vi "TCP_Client.vi"() -> ()   [LabVIEW 2024]
panel:
  in  "Stop Button":bool
  in  "Request":bool
  out "Waveform Graph":dbl[](graph)
  in  "Address":string
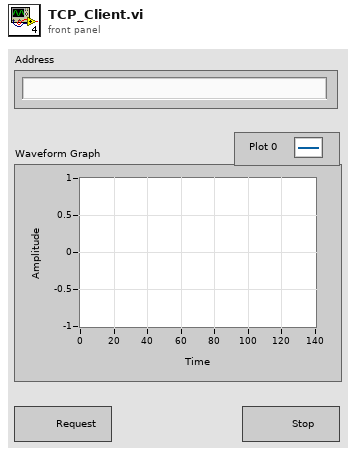
[diagram p1: front panel]
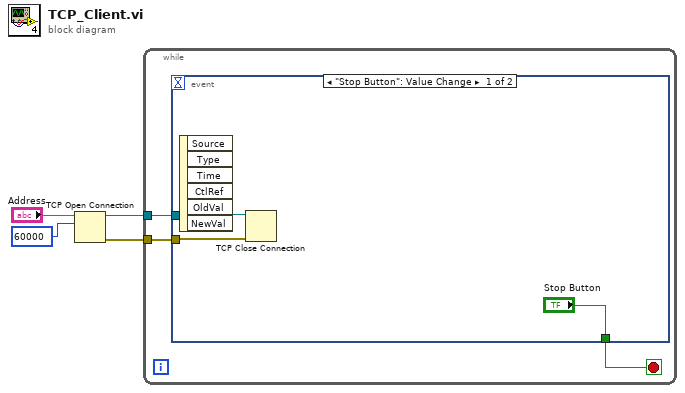
[diagram p0: block diagram]
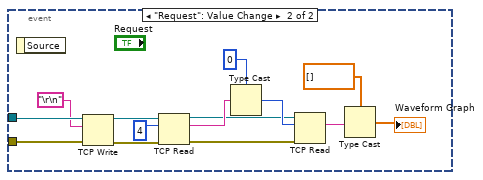
[diagram p2: hidden frame]
diagram:
  n1 = TCP Open Connection(address="Address", remote port or service name=u16 60000) -> (connection ID=w2:refnum<k5>, error out=w1:errorcluster)  [unwired: 3 in]
  n2 = while {
    tunnel: w2 -> [w7]
    tunnel: w1 -> [w6]
    stop <- w5 stop-if-true
    n3 = event shown="[0] \"Stop Button\": Value Change" {
      selector: _ -> [_ _]
      dyn-events: _ -> [_ _]
      timeout: _ -> [_ _]
      tunnel: w7 -> [w9 w24]
      tunnel: w6 -> [w8 w23]
      tunnel: ["Stop Button" _] -> w5
      event "Stop Button": Value Change {
        n4 = event-data() -> ()  [unwired: 1 in, 6 out]
        n5 = TCP Close Connection(connection ID=w9, error in (no error)=w8) -> ()  [unwired: 1 in, 2 out]
      }
      event "Request": Value Change {
        n6 = event-data() -> ()  [unwired: 1 in, 1 out]
        n7 = TCP Write(connection ID=w24, data in="\r\n", error in (no error)=w23) -> (connection ID out=w22:refnum<k5>, error out=w21:errorcluster)  [unwired: 1 in, 1 out]
        n8 = TCP Read(connection ID=w22, bytes to read=4, error in (no error)=w21) -> (connection ID out=w15:refnum<k5>, data out=w17:string, error out=w19:errorcluster)  [unwired: 2 in]
        n9 = Type Cast(type=0, x=w17) -> (*(type *) &x=w16:i32)
        n10 = TCP Read(connection ID=w15, bytes to read=w16, error in (no error)=w19) -> (data out=w13:string)  [unwired: 2 in, 2 out]
        n11 = Type Cast(type=dbl[] [] ("Waveform Graph"), x=w13) -> (*(type *) &x=→"Waveform Graph":dbl[])
      }
    }
  }
